vi "AngeloRTV Snap for imaq.vi"(2 "Image In":T1, 3 "Error_In":i16, 4 "Initialized Array":T2, 5 "PortNo":u16) -> (0 "Error_Out":i16, 1 "Image Out":T1)   [LabVIEW 2012]
uses:
  <vilib>/vision/Image Controls.llb/IMAQ Image.ctl
panel:
  out "error out":errorcluster
  out "bit depth":u8
  out "size(s)":i32[](array[numeric])
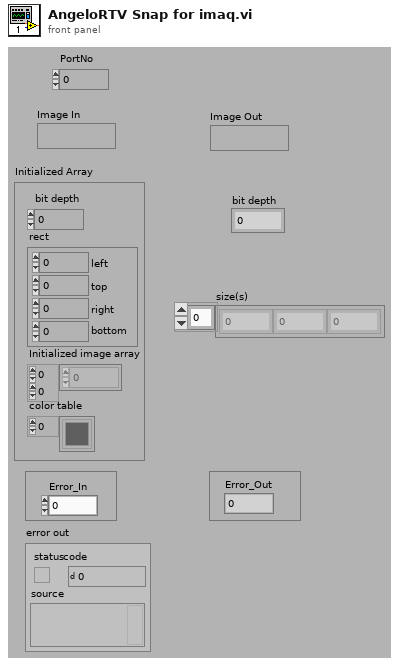
[diagram p1: front panel]
types:
  T1 = typedef "IMAQ Image.ctl" = refnum<image>
  T2 = cluster{"bit depth":u8, "rect":cluster{"left":i16, "top":i16, "right":i16, "bottom":i16}, "Initialized image array":u8[][], "color table":u32[]}
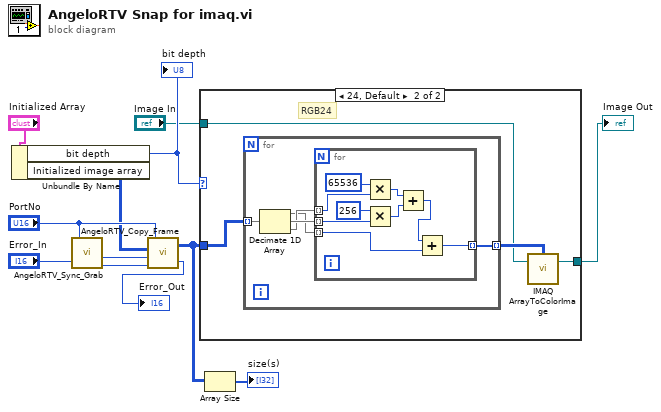
[diagram p0: block diagram]
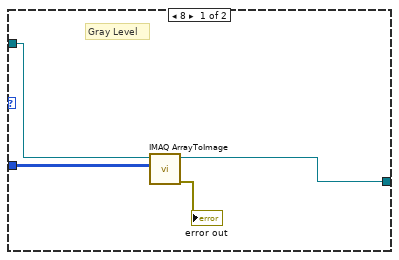
[diagram p2: hidden frame]
diagram:
  n1 = Unbundle By Name("Initialized Array") -> ("bit depth"=w6:u8, "Initialized image array"=w7:u8[][])
  "bit depth" <- w6
  n2 = call "AngeloRTV_Sync_Grab.vi"("Error_In"="Error_In", "PortNo"="PortNo") -> ("Error_Out"=w9:i16, "Szie_Byte"=w10:u32)  [unwired: 3 out]
  n3 = call "AngeloRTV_Copy_Frame.vi"("Error_In"=w9, "Szie_Byte"=w10, "Dest_Addr"=w7, "PortNo"="PortNo") -> ("Error_Out"=→"Error_Out":i16, "Dest_Addr"=w2:u8[][])
  n4 = case shown="24, Default" w6 {
    tunnel: w2 -> [w16 w20]
    tunnel: "Image In" -> [w15 w18]
    tunnel: [w14 w17] -> w3
    frame 8 {
      # "Gray Level"
      n5 = call "IMAQ ArrayToImage"("Image Pixels (U8)"=w16, "Image"=w15) -> ("error out"=→"error out":errorcluster, "Image Out"=w14:T1)  [unwired: 8 in]
    }
    frame 24, Default {
      # "RGB24"
      n6 = for {
        tunnel: w20 -> [w23] mode=indexing
        tunnel: [w22] -> w19 mode=indexing
        n7 = Decimate 1D Array(w23) -> (w21:u8[], w25:u8[], w24:u8[])
        n8 = for {
          tunnel: w25 -> [w31] mode=indexing
          tunnel: w24 -> [w34] mode=indexing
          tunnel: [w26] -> w22 mode=indexing
          tunnel: w21 -> [w27] mode=indexing
          n9 = Multiply(x=u32 65536, y=w34) -> (x*y=w30:u32)
          n10 = Multiply(x=u32 256 ("y"), y=w31) -> (x*y=w29:u32)
          n11 = Add(x=w30, y=w29) -> (x+y=w28:u32)
          n12 = Add(x=w28, y=w27) -> (x+y=w26:u32)
        }
      }
      n13 = call "IMAQ ArrayToColorImage"("Image Pixels (U32)"=w19, "Image"=w18) -> ("Image Out"=w17:T1)  [unwired: 3 in, 1 out]
    }
  }
  "Image Out" <- w3
  n14 = Array Size(array=w2) -> (size(s)=→"size(s)":i32[])
